vi "Voltage to Distance.vi"(2 "error in (no error)":errorcluster, 3 "Voltage":dbl) -> (0 "error out":errorcluster, 1 "Distance":dbl)   [LabVIEW 2015, in "SonarSensor.lvclass"]
uses:
  SonarSensor.lvclass
  SonarSensor.lvclass/SonarSensor.ctl
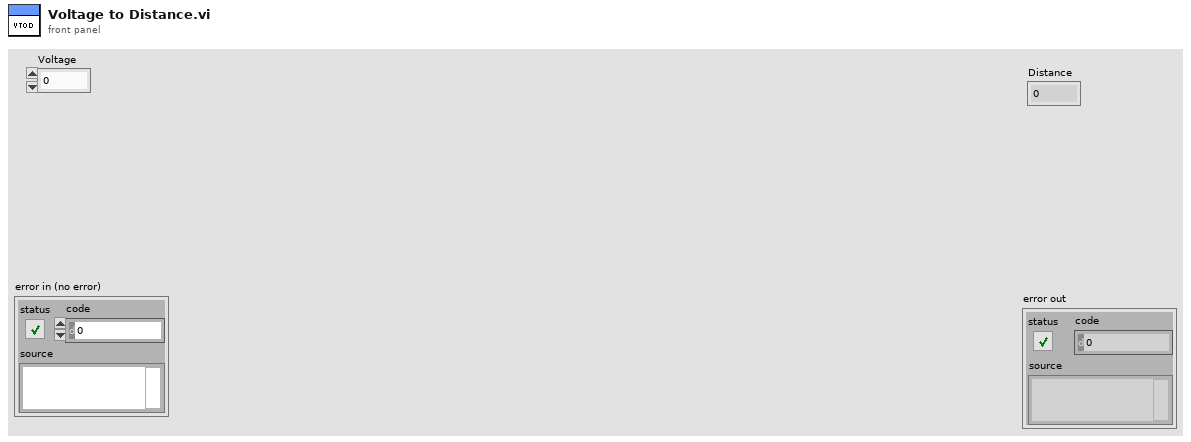
[diagram p1: front panel]
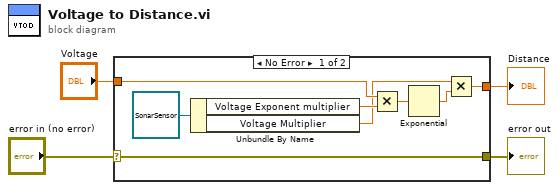
[diagram p0: block diagram]
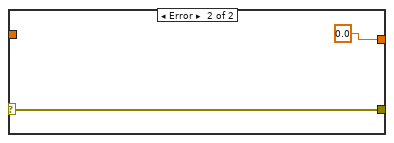
[diagram p2: hidden frame]
diagram:
  n1 = case shown="No Error" "error in (no error)" {
    selector: "error in (no error)" -> [w12 w14]
    tunnel: [w12 w14] -> w3
    tunnel: "Voltage" -> [w9 _]
    tunnel: [w8 0.0] -> w1
    frame No Error {
      n2 = Unbundle By Name(refnum<class "SonarSensor.lvclass"> refnum ("SonarSensor.lvclass")) -> ("Voltage Exponent multiplier"=w6:dbl, "Voltage Multiplier"=w5:dbl)
      n3 = Multiply(x=w9, y=w6) -> (x*y=w10:dbl)
      n4 = Exponential(1:w10) -> (0:w11:dbl)
      n5 = Multiply(x=w5, y=w11) -> (x*y=w8:dbl)
    }
    frame Error {
    }
  }
  "error out" <- w3
  "Distance" <- w1
